vi "Two Path Dummy.vi"(8 "error in (no error)":errorcluster, 11 "Boolean":bool) -> (0 "error out":errorcluster)   [LabVIEW 2020, in "LUnit Tests.lvlib" / "Coverage Test.lvclass"]
uses:
  Coverage Test.lvclass
  Coverage Test.lvclass/Coverage Test.ctl
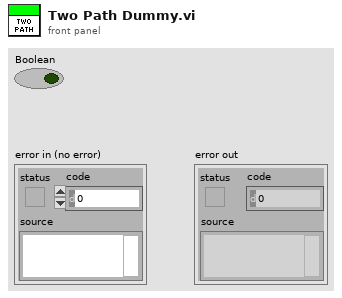
[diagram p1: front panel]
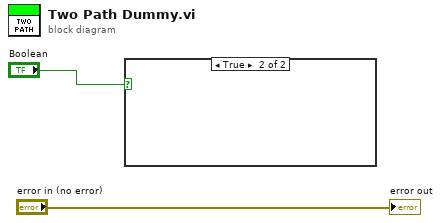
[diagram p0: block diagram]
diagram:
  n1 = case shown="True" "Boolean" {
    frame False {
    }
    frame True {
    }
  }
  "error out" <- "error in (no error)"
